vi "KE6220 -- Set Arm Layer Trig Layer Params.vi"(0 "Resource In":refnum<visa-resource-name>, 1 "Check For SCPI Errors? (T)":bool=TRUE, 7 "6220 Arm Trig Wave Trig Params In":T1={"Arm Layer Input Trig Bypassed?"=FALSE, "Arm Layer Input Trig Source"=enum."Immediate", "Arm Layer Input Trig Link Line"=enum."1", "Arm Layer Input Trig Timer Interval (s)"=0.001, "Arm Layer Output Trig Mode"=enum."No Trig Out", "Arm Layer Output Trig Link Line"=enum."1", "Trig Layer Input Trig Source"=enum."Immediate", "Trig Layer Input Trig Link Line"=enum."1", "Trig Layer Output Trig Mode"=enum."No Trig Out", "Trig Layer Output Trig Link Line"=enum."1"} {"Arm Layer Input Trig Timer Interval (s)" min=0.001 max=99999.999 step=0.001 format="%.3f"}, 11 "error in (no error)":errorcluster) -> (4 "Resource Out (dupl)":refnum<visa-resource-name>, 8 "6220 Arm Trig Wave Trig Params Out":T1={"Arm Layer Input Trig Bypassed?"=FALSE, "Arm Layer Input Trig Source"=enum."Immediate", "Arm Layer Input Trig Link Line"=enum."1", "Arm Layer Input Trig Timer Interval (s)"=0.001, "Arm Layer Output Trig Mode"=enum."No Trig Out", "Arm Layer Output Trig Link Line"=enum."1", "Trig Layer Input Trig Source"=enum."Immediate", "Trig Layer Input Trig Link Line"=enum."1", "Trig Layer Output Trig Mode"=enum."No Trig Out", "Trig Layer Output Trig Link Line"=enum."1"} {"Arm Layer Input Trig Timer Interval (s)" min=0.001 max=99999.999 step=0.001 format="%.3f"}, 15 "error out":errorcluster)   [LabVIEW 2019, in "Keithley 622x.lvlib"]
doc: "Sets the parameters for the 'Arm' and 'Trigger' layers of the trigger model. Note that this VI can be used with both the 6220 and 6221, but it is really intended for use with the 6220, since there is a corresponding VI for the 6221."
uses:
  Keithley 622x.lvlib
  Typedefs/KE6220 -- Arm Trig Params.ctl
  Low Level/Typedefs/KE622x -- Arm Source.ctl
  Low Level/Typedefs/KE622x -- Trig Link Line.ctl
  Low Level/Typedefs/KE622x -- Arm Timer Interval.ctl
  Low Level/Typedefs/KE622x -- Arm Output Mode.ctl
  Low Level/Typedefs/KE622x -- Trig Source.ctl
  Low Level/Typedefs/KE622x -- Trig Output Mode.ctl
panel:
  out "Num Errors":u32
  out "Errors":string[](array[string])
  # "Arm Layer"
  # "Trig Layer"
  # "Arm Layer"
  # "Trig Layer"
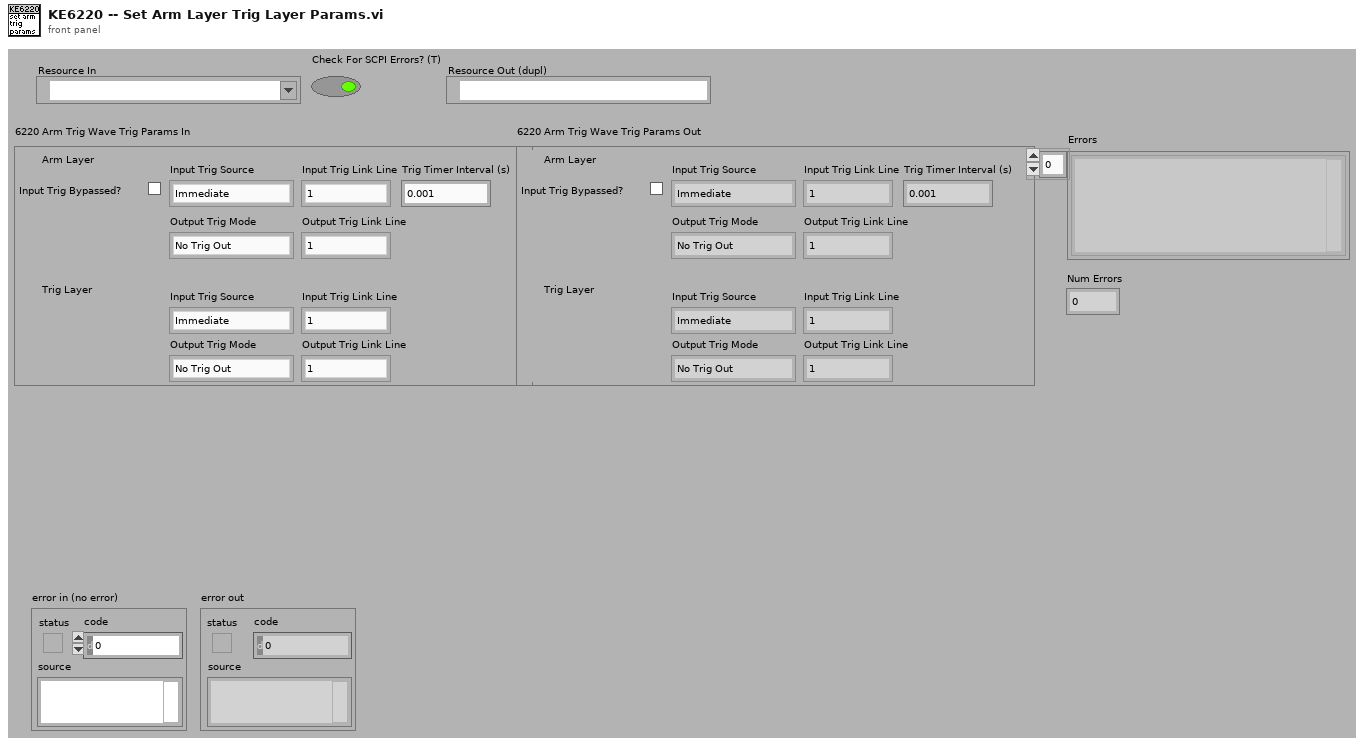
[diagram p1: front panel]
types:
  T1 = typedef "Keithley 622x.lvlib/KE6220 -- Arm Trig Params.ctl" = cluster{"Arm Layer Input Trig Bypassed?":bool, "Arm Layer Input Trig Source":T2, "Arm Layer Input Trig Link Line":T3, "Arm Layer Input Trig Timer Interval (s)":T4, "Arm Layer Output Trig Mode":T5, "Arm Layer Output Trig Link Line":T3, "Trig Layer Input Trig Source":T6, "Trig Layer Input Trig Link Line":T3, "Trig Layer Output Trig Mode":T7, "Trig Layer Output Trig Link Line":T3}
  T2 = typedef "Keithley 622x.lvlib/KE622x -- Arm Source.ctl" = enum16{"Immediate", "Bus (*TRG)", "Timer", "Manual", "Trigger Link", "SOT Falling Edge", "SOT Rising Edge", "SOT Either Edge"}
  T3 = typedef "Keithley 622x.lvlib/KE622x -- Trig Link Line.ctl" = enum16{"1", "2", "3", "4", "5", "6"}
  T4 = typedef "Keithley 622x.lvlib/KE622x -- Arm Timer Interval.ctl" = dbl
  T5 = typedef "Keithley 622x.lvlib/KE622x -- Arm Output Mode.ctl" = enum16{"No Trig Out", "Trig Out On Enter Arm", "Trig Out On Exit Arm"}
  T6 = typedef "Keithley 622x.lvlib/KE622x -- Trig Source.ctl" = enum16{"Immediate", "Trigger Link"}
  T7 = typedef "Keithley 622x.lvlib/KE622x -- Trig Output Mode.ctl" = enum16{"No Trig Out", "Source Turn On", "After Source Delay"}
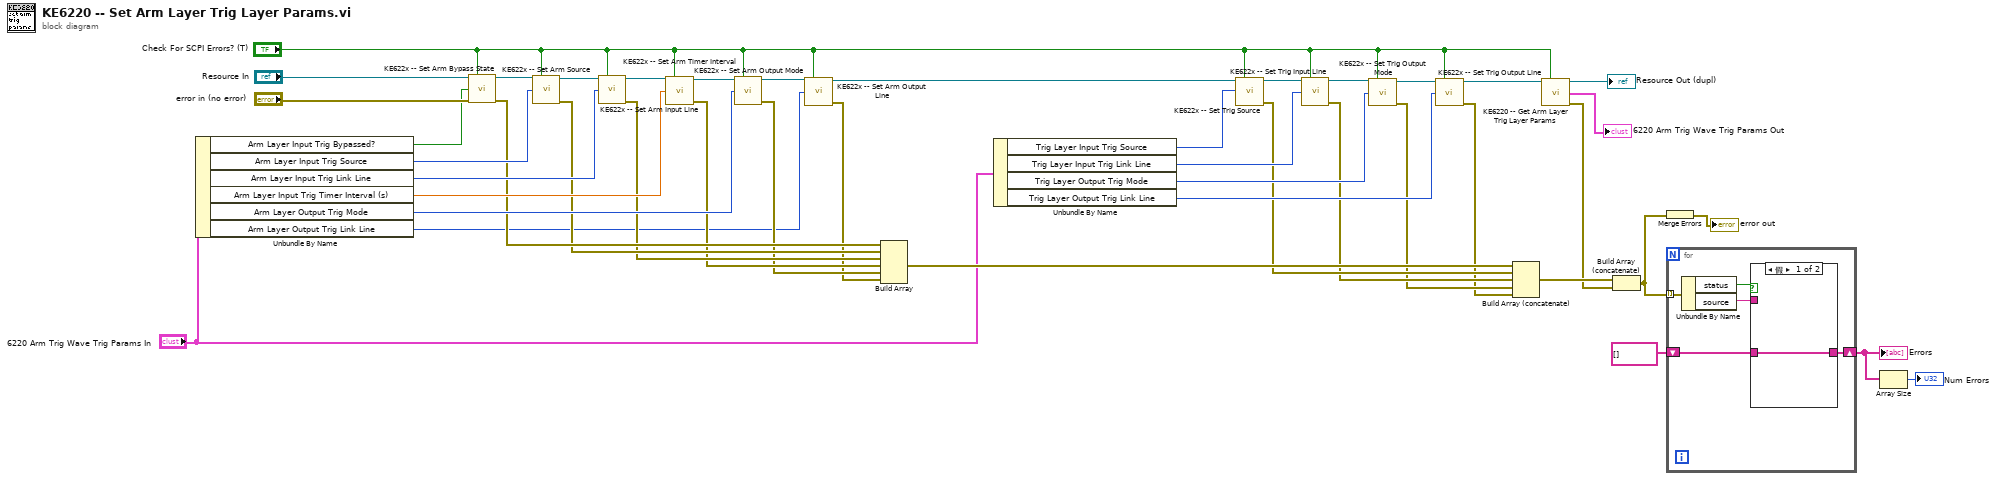
[diagram p0: block diagram]
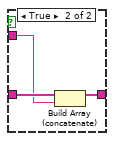
[diagram p2: hidden frame]
diagram:
  n1 = Unbundle By Name("6220 Arm Trig Wave Trig Params In") -> ("Arm Layer Input Trig Bypassed?"=w42:bool, "Arm Layer Input Trig Source"=w40:T2, "Arm Layer Input Trig Link Line"=w38:T3, "Arm Layer Input Trig Timer Interval (s)"=w37:T4, "Arm Layer Output Trig Mode"=w35:T5, "Arm Layer Output Trig Link Line"=w26:T3)
  n2 = call "KE622x -- Set Arm Bypass State.vi"("Resource In"="Resource In", "Check For SCPI Errors? (T)"="Check For SCPI Errors? (T)", "Bypass Arm Layer?"=w42, "error in (no error)"="error in (no error)") -> ("Resource Out (dupl)"=w39:refnum<visa-resource-name>, "error out"=w32:errorcluster)  [unwired: 10 in]
  n3 = call "KE622x -- Set Arm Source.vi"("Resource In"=w39, "Check For SCPI Errors? (T)"="Check For SCPI Errors? (T)", "Arm Source"=w40) -> ("Resource Out (dupl)"=w41:refnum<visa-resource-name>, "error out"=w31:errorcluster)  [unwired: 11 in]
  n4 = call "KE622x -- Set Arm Input Line.vi"("Resource In"=w41, "Check For SCPI Errors? (T)"="Check For SCPI Errors? (T)", "Arm Input Line"=w38) -> ("Resource Out (dupl)"=w36:refnum<visa-resource-name>, "error out"=w30:errorcluster)  [unwired: 11 in]
  n5 = call "KE622x -- Set Arm Timer Interval.vi"("Resource In"=w36, "Check For SCPI Errors? (T)"="Check For SCPI Errors? (T)", "Arm Timer Interval (s)"=w37) -> ("Resource Out (dupl)"=w34:refnum<visa-resource-name>, "error out"=w29:errorcluster)  [unwired: 10 in, 1 out]
  n6 = call "KE622x -- Set Arm Output Mode.vi"("Resource In"=w34, "Check For SCPI Errors? (T)"="Check For SCPI Errors? (T)", "Arm Output Mode"=w35) -> ("Resource Out (dupl)"=w33:refnum<visa-resource-name>, "error out"=w28:errorcluster)  [unwired: 11 in]
  n7 = call "KE622x -- Set Arm Output Line.vi"("Resource In"=w33, "Check For SCPI Errors? (T)"="Check For SCPI Errors? (T)", "Arm Output Line"=w26) -> ("Resource Out (dupl)"=w25:refnum<visa-resource-name>, "error out"=w27:errorcluster)  [unwired: 11 in]
  n8 = Build Array(w32, w31, w30, w29, w28, w27) -> (w17:errorcluster[])
  n9 = Unbundle By Name("6220 Arm Trig Wave Trig Params In") -> ("Trig Layer Input Trig Source"=w24:T6, "Trig Layer Input Trig Link Line"=w22:T3, "Trig Layer Output Trig Mode"=w20:T7, "Trig Layer Output Trig Link Line"=w19:T3)
  n10 = call "KE622x -- Set Trig Source.vi"("Resource In"=w25, "Check For SCPI Errors? (T)"="Check For SCPI Errors? (T)", "Trig Source"=w24) -> ("Resource Out (dupl)"=w23:refnum<visa-resource-name>, "error out"=w16:errorcluster)  [unwired: 11 in]
  n11 = call "KE622x -- Set Trig Input Line.vi"("Resource In"=w23, "Check For SCPI Errors? (T)"="Check For SCPI Errors? (T)", "Trig Input Line"=w22) -> ("Resource Out (dupl)"=w21:refnum<visa-resource-name>, "error out"=w15:errorcluster)  [unwired: 11 in]
  n12 = call "KE622x -- Set Trig Output Mode.vi"("Resource In"=w21, "Check For SCPI Errors? (T)"="Check For SCPI Errors? (T)", "Trig Output Mode"=w20) -> ("Resource Out (dupl)"=w18:refnum<visa-resource-name>, "error out"=w14:errorcluster)  [unwired: 11 in]
  n13 = call "KE622x -- Set Trig Output Line.vi"("Resource In"=w18, "Check For SCPI Errors? (T)"="Check For SCPI Errors? (T)", "Trig Output Line"=w19) -> ("Resource Out (dupl)"=w3:refnum<visa-resource-name>, "error out"=w13:errorcluster)  [unwired: 11 in]
  n14 = Build Array (concatenate)(w17, w16, w15, w14, w13) -> (w4:errorcluster[])
  n15 = call "KE6220 -- Get Arm Layer Trig Layer Params.vi"("Resource In"=w3, "Check For SCPI Errors? (T)"="Check For SCPI Errors? (T)") -> ("Resource Out (dupl)"=→"Resource Out (dupl)":refnum<visa-resource-name>, "6220 Arm Trig Params"=→"6220 Arm Trig Wave Trig Params Out":T1, "error out"=w1:errorcluster)  [unwired: 11 in]
  n16 = Build Array (concatenate)(w4, w1) -> (w9:errorcluster[])
  n17 = Merge Errors(w9) -> (→"error out":errorcluster)
  n18 = for {
    tunnel: w9 -> [w49] mode=indexing
    shift-right: [w45] -> w6
    shift-left: string[] [] -> [w46]
    n19 = Unbundle By Name(w49) -> ("status"=w48:bool, "source"=w47:string)
    n20 = case shown="假" w48 {
      tunnel: w47 -> [_ w52]
      tunnel: w46 -> [w50 w53]
      tunnel: [w50 w51] -> w45
      frame False {
      }
      frame True {
        n21 = Build Array (concatenate)(w53, w52) -> (w51:string[])
      }
    }
  }
  "Errors" <- w6
  n22 = Array Size(array=w6) -> (size(s)=→"Num Errors":i32)
